vi "Read reg control.vi"(8 "error in (no error)":errorcluster, 10 "value":string, 11 "HT_in in":T1 {"Y_H" step=1.0; "SP" step=0.01 format="%.2f"}) -> (0 "error out":errorcluster, 2 "Data to Write":bool, 3 "HT1_in out":T1 {"Y_H" step=1.0; "SP" step=0.01 format="%.2f"})   [LabVIEW 2019, in "OPC addons.lvlib"]
uses:
  OPC addons.lvlib
  Reg/ctl/ZY_control_short.ctl
  Reg/ctl/Z_State.ctl
  Reg/ctl/Y_state.ctl
  <vilib>/JDP Science/JSONtext/String Subset.vi
  <vilib>/JDP Science/JSONtext/support/Strip Quotes and Unescape.vi
  <vilib>/JDP Science/JSONtext/Parsing/Parse Full Path or Item Name.vi
  <vilib>/JDP Science/JSONtext/Offset/Find Item Locations by Path.vi
  <vilib>/JDP Science/JSONtext/support/Unescape JSON string.vi
  <vilib>/JDP Science/JSONtext/JSONtext.lvlib
  Reg/control.lvlib
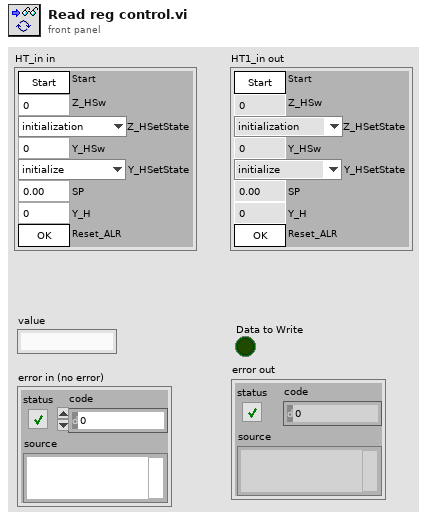
[diagram p1: front panel]
types:
  T1 = typedef "control.lvlib/ZY_control_short.ctl" = cluster{"Start":bool, "Z_HSw":u32, "Z_HSetState":T2, "Y_HSw":u32, "Y_HSetState":T3, "SP":dbl, "Y_H":dbl, "Reset_ALR":bool}
  T2 = typedef "control.lvlib/Z_State.ctl" = enum8{"initialization", "alarm", "disabled", "not ready", "stop ready", "reserv", "switched off", "reserv2", "switched on", "check", "on min", "decrease out", "on", "increase out", "on max"}
  T3 = typedef "control.lvlib/Y_state.ctl" = enum8{"initialize", "alarm", "min", "stop", "hand", "auto", "max"}
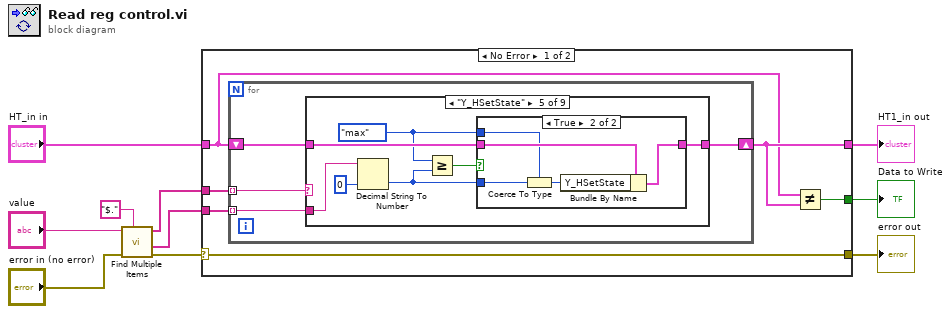
[diagram p0: block diagram]
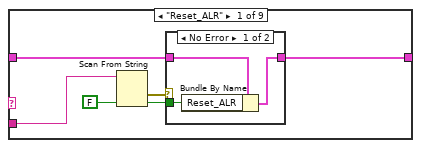
[diagram p2: hidden frame]
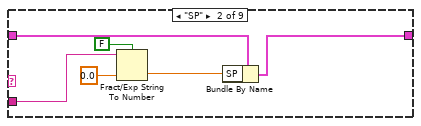
[diagram p4: hidden frame]
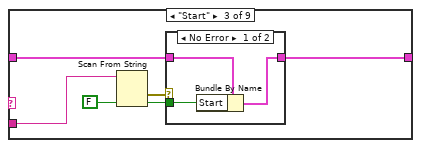
[diagram p5: hidden frame]
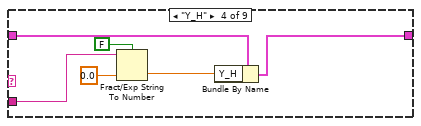
[diagram p7: hidden frame]
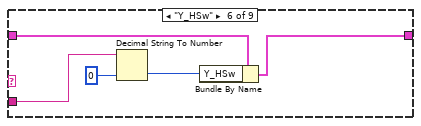
[diagram p9: hidden frame]
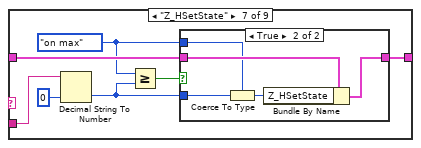
[diagram p10: hidden frame]
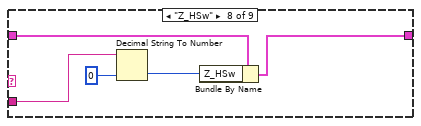
[diagram p12: hidden frame]
diagram:
  n1 = call <vilib>:"Find Multiple Items.vi"("$Path or Item Name"="$.", "error in (no error)"="error in (no error)", "JSON"="value") -> ("error out"=w7:errorcluster, "<JSON>"=w5:string[], "Item Names"=w10:string[])  [unwired: 5 in, 1 out]
  n2 = case shown="No Error" w7 {
    selector: w7 -> [w13 w90]
    tunnel: w10 -> [w16 _]
    tunnel: "HT_in in" -> [w11 w91]
    tunnel: w5 -> [w15 _]
    tunnel: [w12 w91] -> w6
    tunnel: [w14 _] -> w2
    tunnel: [w13 w90] -> w1
    frame No Error {
      n3 = for {
        shift-right: [w18] -> w12
        shift-left: w11 -> [w20]
        tunnel: w16 -> [w17] mode=indexing
        tunnel: w15 -> [w19] mode=indexing
        n4 = case shown="\"Y_HSetState\"" w17 {
          tunnel: w20 -> [w26 w36 w42 w52 w59 w70 w77 w88 w89]
          tunnel: w19 -> [w23 w33 w39 w49 w57 w67 w75 w85 _]
          tunnel: [w25 w32 w41 w48 w56 w66 w74 w84 w89] -> w18
          frame "Reset_ALR" {
            n5 = Scan From String(input string=w23, default 1=FALSE ("use system decimal point (T)")) -> (error out=w21:errorcluster, output 1=w22:bool)  [unwired: 3 in, 2 out]
            n6 = case shown="No Error" w21 {
              tunnel: w26 -> [w29 w30]
              tunnel: [w28 w30] -> w25
              tunnel: w22 -> [w27 _]
              frame No Error {
                n7 = Bundle By Name(cluster=w29, "Reset_ALR"=w27) -> (w28:T1)
              }
              frame Error {
              }
            }
          }
          frame "SP" {
            n8 = Fract/Exp String To Number(use system decimal point (T)=FALSE, string=w33, default (0 dbl)=0.0 ("Z_HSw")) -> (number=w34:dbl)  [unwired: 1 in, 1 out]
            n9 = Bundle By Name(cluster=w36, "SP"=w34) -> (w32:T1)
          }
          frame "Start" {
            n10 = Scan From String(input string=w39, default 1=FALSE ("use system decimal point (T)")) -> (error out=w37:errorcluster, output 1=w38:bool)  [unwired: 3 in, 2 out]
            n11 = case shown="No Error" w37 {
              tunnel: w42 -> [w45 w46]
              tunnel: [w44 w46] -> w41
              tunnel: w38 -> [w43 _]
              frame No Error {
                n12 = Bundle By Name(cluster=w45, "Start"=w43) -> (w44:T1)
              }
              frame Error {
              }
            }
          }
          frame "Y_H" {
            n13 = Fract/Exp String To Number(use system decimal point (T)=FALSE, string=w49, default (0 dbl)=0.0 ("Z_HSw")) -> (number=w50:dbl)  [unwired: 1 in, 1 out]
            n14 = Bundle By Name(cluster=w52, "Y_H"=w50) -> (w48:T1)
          }
          frame "Y_HSetState" {
            w53 = Y_state."max" ("Y_HSetState")
            n15 = Decimal String To Number(string=w57, default (0L)=u8 0 ("Z_HSw")) -> (number=w54:u8)  [unwired: 1 in, 1 out]
            n16 = Greater Or Equal?(x=w53, y=w54) -> (x >= y?=w55:bool)
            n17 = case shown="True" w55 {
              tunnel: w59 -> [w60 w65]
              tunnel: [w60 w64] -> w56
              tunnel: w53 -> [_ w62]
              tunnel: w54 -> [_ w61]
              frame False {
              }
              frame True {
                n18 = Coerce To Type(0:w61, 1:w62) -> (2:w63:T3)
                n19 = Bundle By Name(cluster=w65, "Y_HSetState"=w63) -> (w64:T1)
              }
            }
          }
          frame "Y_HSw" {
            n20 = Decimal String To Number(string=w67, default (0L)=u32 0 ("Z_HSw")) -> (number=w68:u32)  [unwired: 1 in, 1 out]
            n21 = Bundle By Name(cluster=w70, "Y_HSw"=w68) -> (w66:T1)
          }
          frame "Z_HSetState" {
            w73 = Z_State."on max" ("Z_HSetState")
            n22 = Decimal String To Number(string=w75, default (0L)=u8 0 ("Z_HSw")) -> (number=w71:u8)  [unwired: 1 in, 1 out]
            n23 = Greater Or Equal?(x=w73, y=w71) -> (x >= y?=w72:bool)
            n24 = case shown="True" w72 {
              tunnel: w77 -> [w78 w83]
              tunnel: [w78 w82] -> w74
              tunnel: w73 -> [_ w80]
              tunnel: w71 -> [_ w79]
              frame False {
              }
              frame True {
                n25 = Coerce To Type(0:w79, 1:w80) -> (2:w81:T2)
                n26 = Bundle By Name(cluster=w83, "Z_HSetState"=w81) -> (w82:T1)
              }
            }
          }
          frame "Z_HSw" {
            n27 = Decimal String To Number(string=w85, default (0L)=u32 0 ("Z_HSw")) -> (number=w86:u32)  [unwired: 1 in, 1 out]
            n28 = Bundle By Name(cluster=w88, "Z_HSw"=w86) -> (w84:T1)
          }
          frame Default {
          }
        }
      }
      n29 = Not Equal?(x=w11, y=w12) -> (x != y?=w14:bool)
    }
    frame Error {
    }
  }
  "HT1_in out" <- w6
  "Data to Write" <- w2
  "error out" <- w1
